vi "Coordinate_Trans_.vi"(0 "Traverse Name":string, 1 "Input Position":dbl[](array[numeric])=[0.0, 0.0, 0.0] format="%.2f") -> (2 "X":dbl, 3 "Y":dbl, 4 "Z":dbl)   [LabVIEW 2011]
uses:
  Globals/Trav_pos_global.vi
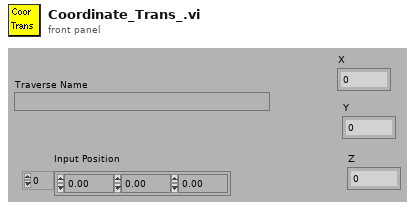
[diagram p1: front panel]
types:
  T1 = typedef "Tunnel_Coordinates.ctl" = enum16{"Work in Tunnel Coordinates", "Work in Model Coordinates"}
  T2 = enum16{"To Traverse Coordinates", "To User Coordinates"}
  T3 = cluster{"Output Position[0]":dbl, "Output Position[1]":dbl, "Output Position[2]":dbl}
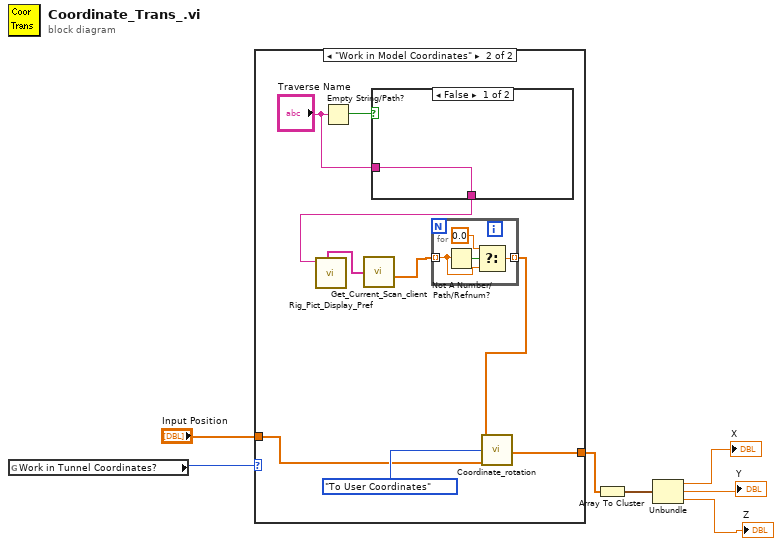
[diagram p0: block diagram]
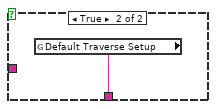
[diagram p3: hidden frame]
diagram:
  n1 = global read "Trav_pos_global.vi" "Work in Tunnel Coordinates?"() -> (w6:T1)
  n2 = case shown="\"Work in Model Coordinates\"" w6 {
    tunnel: [w8 w15] -> w4
    tunnel: "Input Position" -> [w8 w16]
    frame "Work in Tunnel Coordinates" {
    }
    frame "Work in Model Coordinates" {
      n3 = Empty String/Path?(string/path="Traverse Name") -> (empty?=w11:bool)
      n4 = case shown="False" w11 {
        tunnel: [w18 w19] -> w10
        tunnel: "Traverse Name" -> [w18 _]
        frame False {
        }
        frame True {
          n5 = global read "Trav_pos_global.vi" "Default Traverse Setup"() -> (w19:string)
        }
      }
      n6 = call "Rig_Pict_Display_Pref.vi"("Traverse Name"=w10) -> ("Roll Pitch Yaw ADAM Channels"=w14:string[])  [unwired: 3 in, 4 out]
      n7 = call "Get_Current_Scan_client.vi"("ADAM Ch Names"=w14) -> ("Numerical Values"=w13:dbl[])  [unwired: 3 out]
      n8 = for {
        tunnel: w13 -> [w22] mode=indexing
        tunnel: [w20] -> w12 mode=indexing
        n9 = Not A Number/Path/Refnum?(number/path/refnum=w22) -> (NaN/Path/Refnum?=w23:bool)
        n10 = Select(t=0.0, s=w23, f=w22) -> (s? t:f=w20:dbl)
      }
      n11 = call "Coordinate_rotation.vi"("Model       Roll      Pitch       Yaw (deg)"=w12, "Input Position"=w16, "Mode"=T2."To User Coordinates") -> ("Output Position"=w15:dbl[])  [unwired: 2 in, 1 out]
    }
  }
  n12 = Array To Cluster(array=w4) -> (cluster=w5:T3)
  n13 = Unbundle(w5) -> ("Output Position[0]"=→"X":dbl, "Output Position[1]"=→"Y":dbl, "Output Position[2]"=→"Z":dbl)
